vi "Cut_Out_Unsigned_Tracks-1.vi"(0 "[IN] Tracks":dbl[][](array[numeric]), 1 "[IN] Dot Status":i16[][](array[numeric]), 5 "[IN] Start Pos":i32[](array[numeric]), 9 "[IN] Position \nof Mistakes":i32[](array[numeric]), 11 "error IN":errorcluster, 13 "[IN] Track ID":u16[](array[numeric])) -> (3 "[OUT] Dot Status":i16[][](array[numeric]), 4 "[OUT] Tracks":dbl[][](array[numeric]), 6 "[OUT] Track ID":u16[](array[numeric]), 8 "[OUT] Start Pos":i32[](array[numeric]), 10 "[OUT] Missed tracks":dbl[][](array[numeric]), 12 "[OUT] Missed Start Pos":i32[](array[numeric]), 14 "[OUT] Missed Dot Status":i16[][](array[numeric]), 15 "error OUT":errorcluster)   [LabVIEW 2013]
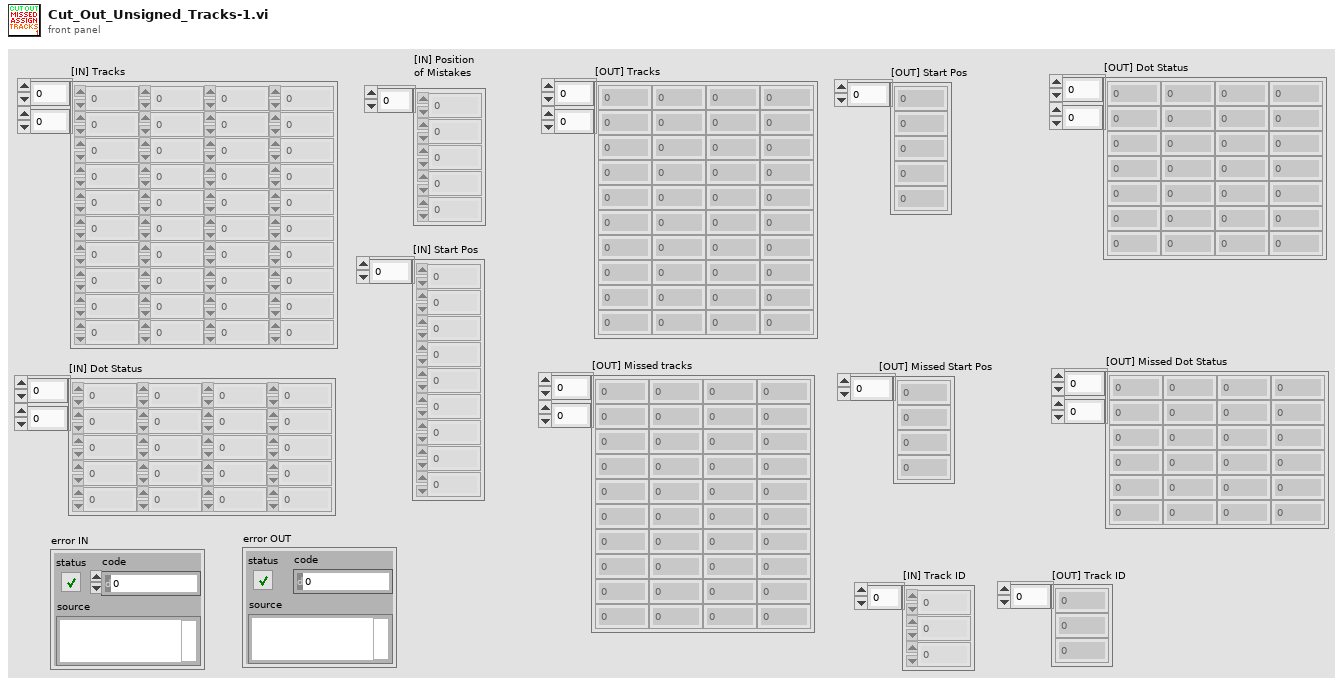
[diagram p1: front panel]
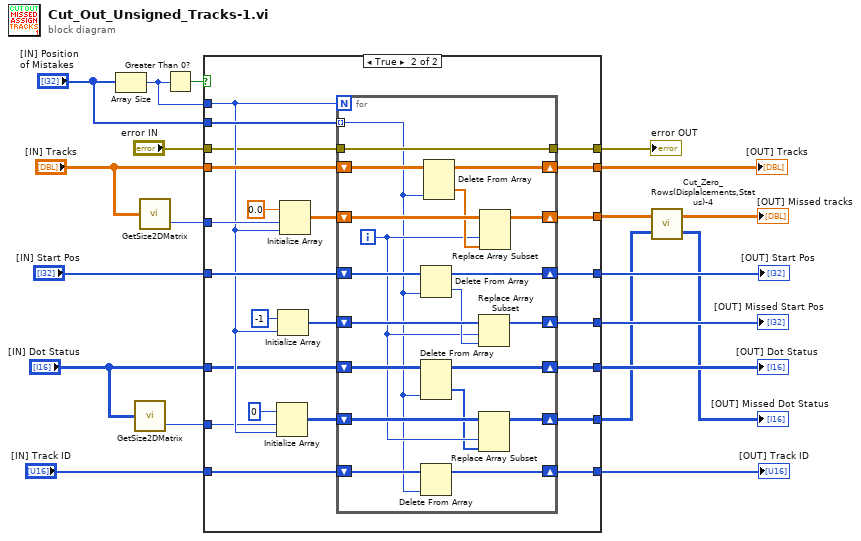
[diagram p0: block diagram]
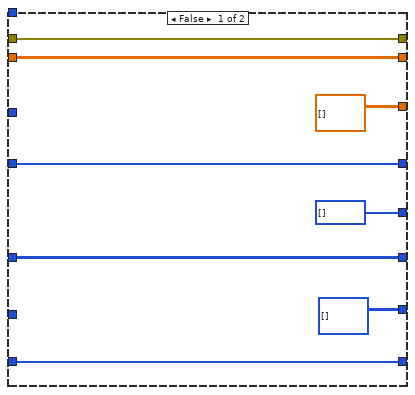
[diagram p2: hidden frame]
diagram:
  n1 = Array Size(array="[IN] Position \nof Mistakes") -> (size(s)=w19:i32)
  n2 = call "GetSize2DMatrix.vi"("Array IN (2D)"="[IN] Dot Status") -> ("# Rows"=w13:i32)  [unwired: 1 out]
  n3 = call "GetSize2DMatrix.vi"("Array IN (2D)"="[IN] Tracks") -> ("# Rows"=w17:i32)  [unwired: 1 out]
  n4 = Greater Than 0?(x=w19) -> (x > 0?=w20:bool)
  n5 = case shown="True" w20 {
    tunnel: w19 -> [_ w43]
    tunnel: "[IN] Position \nof Mistakes" -> [_ w50]
    tunnel: w17 -> [_ w49]
    tunnel: "[IN] Tracks" -> [w26 w48]
    tunnel: "[IN] Start Pos" -> [w27 w45]
    tunnel: "[IN] Dot Status" -> [w25 w41]
    tunnel: w13 -> [_ w40]
    tunnel: "error IN" -> [w28 w38]
    tunnel: [w28 w37] -> w11
    tunnel: [w26 w36] -> w10
    tunnel: [dbl[][] [] w35] -> w7
    tunnel: [w27 w34] -> w9
    tunnel: [i32[] [] w33] -> w5
    tunnel: [w25 w32] -> w8
    tunnel: [i16[][] [] w31] -> w4
    tunnel: "[IN] Track ID" -> [w21 w30]
    tunnel: [w21 w29] -> w1
    frame False {
    }
    frame True {
      n6 = Initialize Array(i16 0, w40, w43) -> (w39:i16[][])
      n7 = Initialize Array(-1, w43) -> (w44:i32[])
      n8 = Initialize Array(0.0 ("element"), w49, w43) -> (w47:dbl[][])
      n9 = for {
        N: w43 -> [_]
        tunnel: w50 -> [w52] mode=indexing
        shift-right: [w64] -> w36
        shift-left: w48 -> [w71]
        shift-right: [w55] -> w35
        shift-left: w47 -> [w70]
        shift-right: [w65] -> w34
        shift-left: w45 -> [w68]
        shift-right: [w57] -> w33
        shift-left: w44 -> [w67]
        shift-right: [w58] -> w32
        shift-left: w41 -> [w63]
        shift-right: [w59] -> w31
        shift-left: w39 -> [w62]
        tunnel: w38 -> [w56]
        tunnel: [w56] -> w37
        shift-right: [w53] -> w29
        shift-left: w30 -> [w54]
        i -> [w61]
        n10 = Delete From Array(array=w68, index=w52) -> (deleted portion=w66:i32, array with subset deleted=w65:i32[])  [unwired: 1 in]
        n11 = Delete From Array(array=w63, index (col)=w52) -> (deleted portion=w60:i16[], array with subset deleted=w58:i16[][])  [unwired: 2 in]
        n12 = Delete From Array(array=w54, index=w52) -> (array with subset deleted=w53:u16[])  [unwired: 1 in, 1 out]
        n13 = Delete From Array(array=w71, index (col)=w52) -> (deleted portion=w69:dbl[], array with subset deleted=w64:dbl[][])  [unwired: 2 in]
        n14 = Replace Array Subset(array=w67, new element=w66, index=w61) -> (w57:i32[])
        n15 = Replace Array Subset(array=w62, new element=w60, index (col)=w61) -> (w59:i16[][])  [unwired: 1 in]
        n16 = Replace Array Subset(array=w70, new element=w69, index (col)=w61) -> (w55:dbl[][])  [unwired: 1 in]
      }
    }
  }
  "error OUT" <- w11
  "[OUT] Tracks" <- w10
  "[OUT] Start Pos" <- w9
  "[OUT] Dot Status" <- w8
  "[OUT] Missed Start Pos" <- w5
  "[OUT] Track ID" <- w1
  n17 = call "Cut_Zero_Rows(Displalcements,Status)-4.vi"("[IN] Dot matrix\nwith zero points"=w4, "[IN] (X,Y,dX,dY) \nwith zero displ"=w7) -> ("[OUT] Dot \nMatrix"=→"[OUT] Missed Dot Status":i16[][], "[OUT] (X,Y,dX,dY)\nw/t zero displac"=→"[OUT] Missed tracks":dbl[][])
